vi "Resize Tree.vi"(0 "Tree Ref":refnum<vi>) -> ()   [LabVIEW 2011, in "VariantXControl__VP.xctl"]
uses:
  VariantXControl__VP.xctl
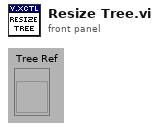
[diagram p1: front panel]
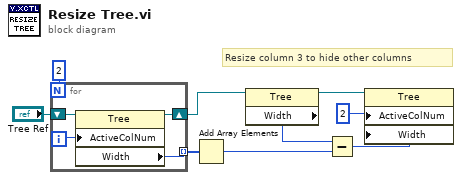
[diagram p0: block diagram]
diagram:
  # "Resize column 3 to hide other columns"
  n1 = for {
    N: 2 -> [_]
    tunnel: [w12] -> w2 mode=indexing
    shift-right: [w10] -> w8
    shift-left: "Tree Ref" -> [w11]
    i -> [w13]
    n2 = property on="Property Node" class="Tree"(reference=w11, "ActiveColNum"=w13) -> (reference out=w10:refnum<vi>, "Width"=w12:i32)  [unwired: 1 in, 1 out]
  }
  n3 = Add Array Elements(numeric array=w2) -> (sum=w7:i32)
  n4 = property on="Property Node" class="Tree"(reference=w8) -> (reference out=w3:refnum<vi>, "Width"=w5:u32)  [unwired: 1 in, 1 out]
  n5 = Subtract(x=w5, y=w7) -> (x-y=w6:u32)
  n6 = property on="Property Node" class="Tree"(reference=w3, "ActiveColNum"=2 ("Active Cell:Active Column Number"), "Width"=w6) -> ()  [unwired: 1 in, 2 out]
